vi "NM TO V CONVERTER.vi"(8 "error in (no error)":errorcluster, 10 "Max Banco":dbl, 11 "Set Point":dbl) -> (0 "error out":errorcluster, 3 "Set Value to cDAQ":dbl)   [LabVIEW 2019]
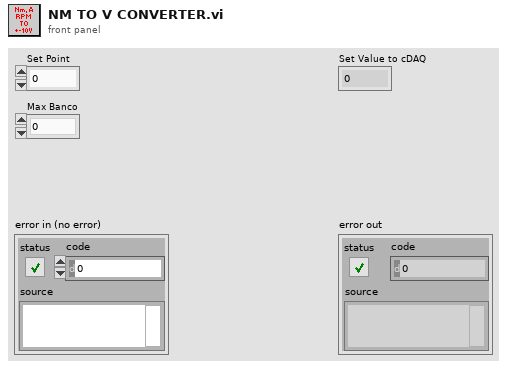
[diagram p1: front panel]
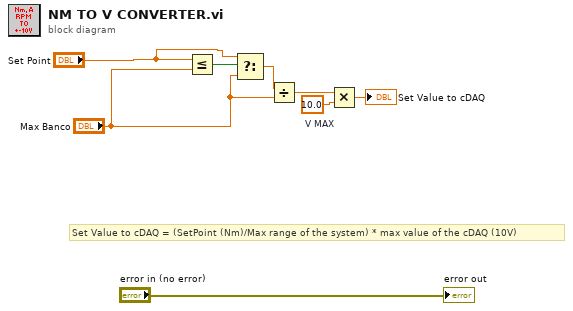
[diagram p0: block diagram]
diagram:
  w7 = 10.0  # V MAX
  # "Set Value to cDAQ = (SetPoint (Nm)/Max range of the system) * max value of the cDAQ (10V)"
  n1 = Less Or Equal?(x="Set Point", y="Max Banco") -> (x <= y?=w4:bool)
  n2 = Select(t="Set Point", s=w4, f="Max Banco") -> (s? t:f=w3:dbl)
  n3 = Divide(x=w3, y="Max Banco") -> (x/y=w8:dbl)
  n4 = Multiply(x=w8, y=w7) -> (x*y=→"Set Value to cDAQ":dbl)
  "error out" <- "error in (no error)"
